vi "ServerVI.vi"() -> ()   [LabVIEW 2021]
uses:
  Resources/ServerEnum.ctl
  <vilib>/Utility/error.llb/DialogType.ctl
  <vilib>/Utility/file.llb/Read Delimited Spreadsheet (string).vi
  <vilib>/Utility/file.llb/Write Delimited Spreadsheet (string).vi
panel:
  in  "CarWashRecord":enum32{"Car Wash Record", "Revenue"}(tab)
  in  "btnLogout":bool
  out "Car Wash Record":string[][](table)
  out "Deluxe":dbl
  out "Economy":dbl
  in  "btnGenerate":bool
  out "Date":string
  out "Revenue ($)":dbl
  in  "LoginTab":enum32{"Login"}(tab)
  in  "Username":string
  in  "Password":string
  in  "btnLogin":bool
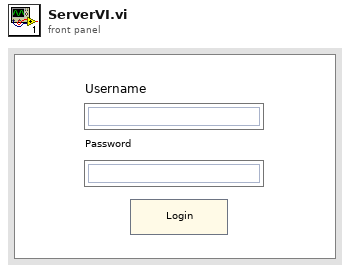
[diagram p1: front panel]
types:
  T1 = typedef "DialogType.ctl" = u16
  T2 = typedef "ServerEnum.ctl" = enum16{"Initialization", "Setup", "Validation", "ShowUI", "Format", "Error"}
  T3 = enum8{"Enabled", "Disabled", "Disabled and Grayed Out"}
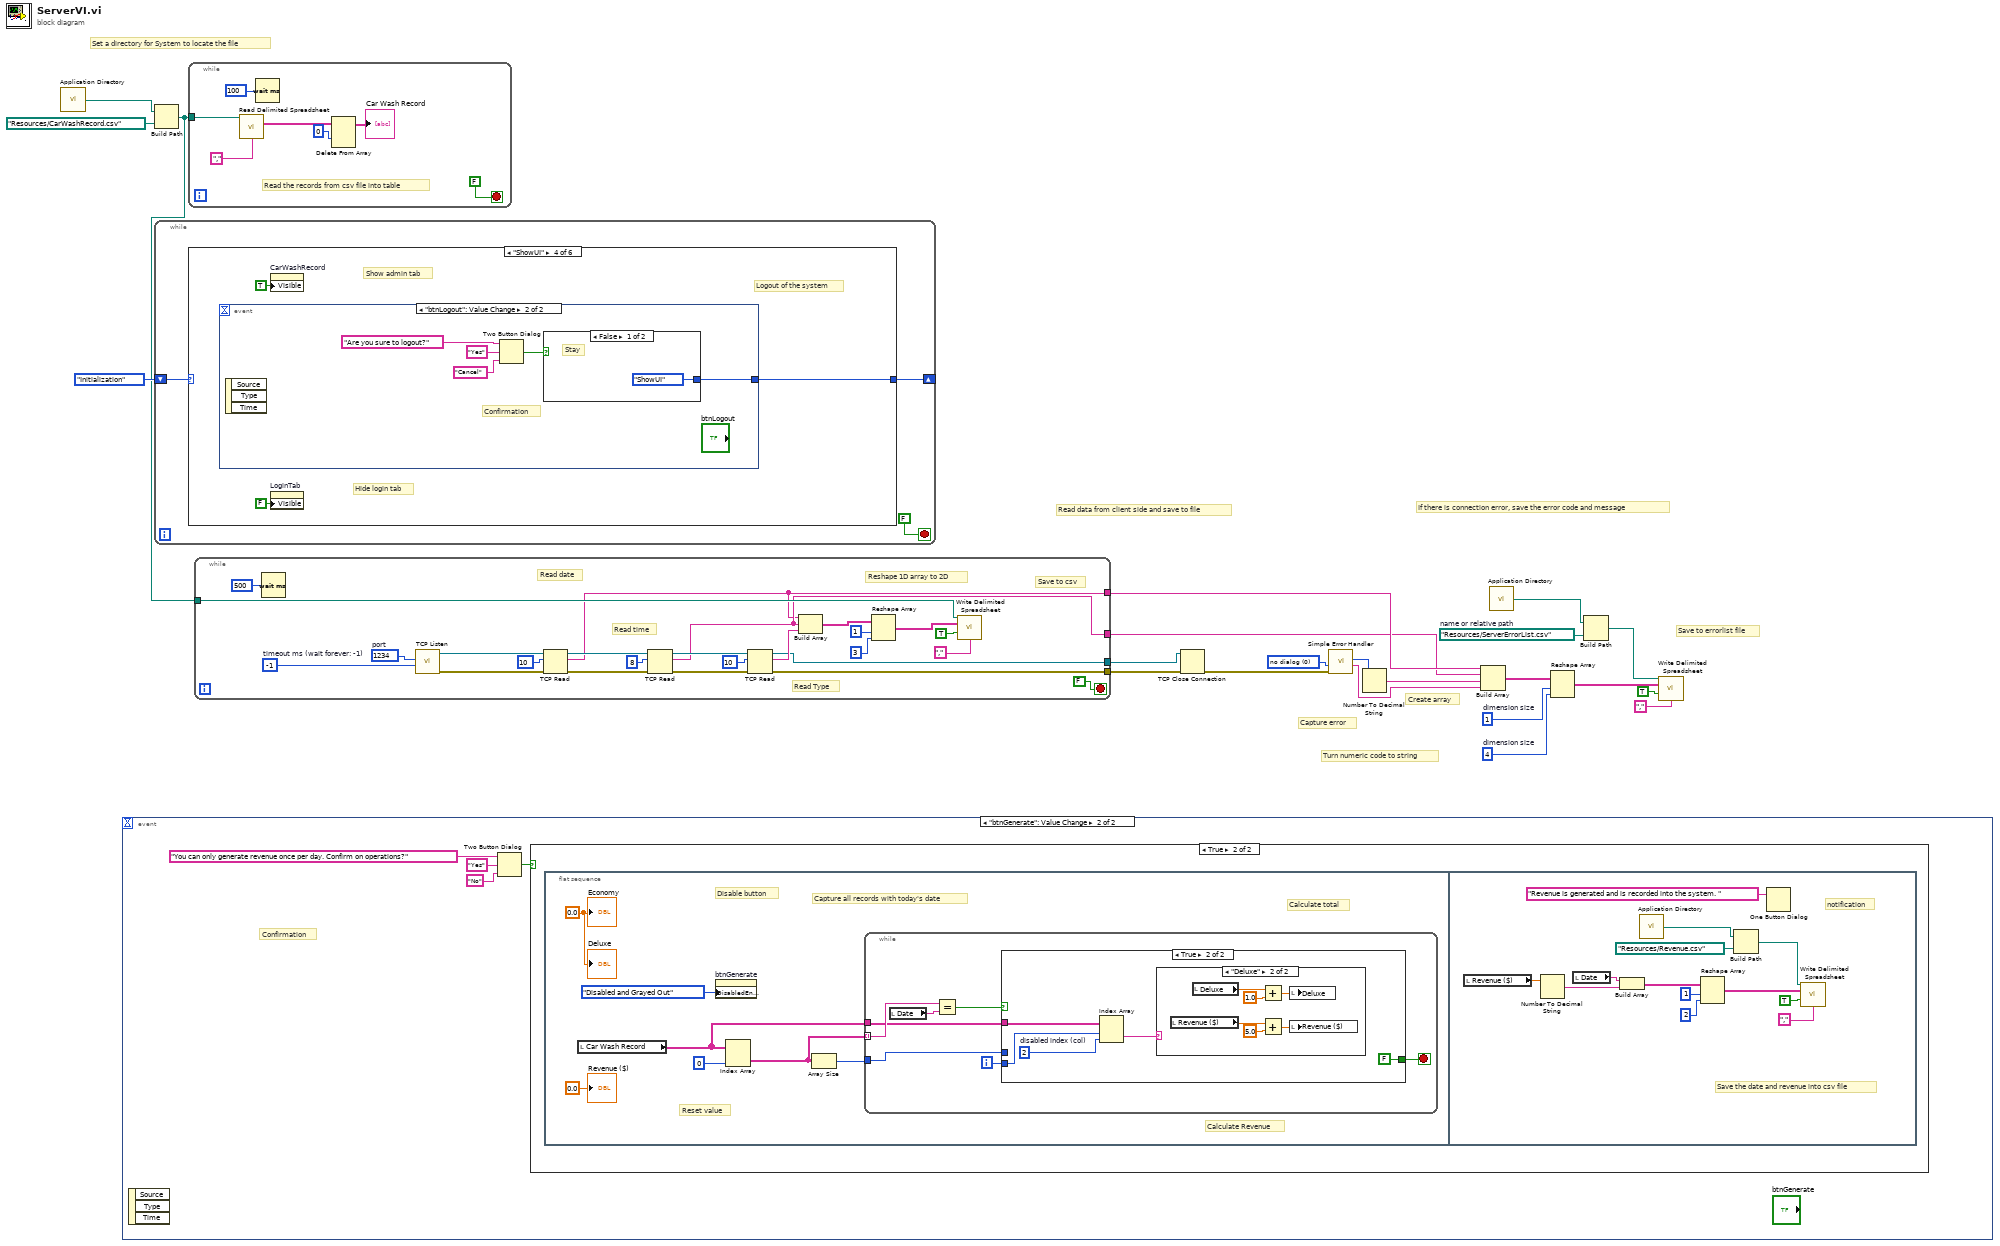
[diagram p0: block diagram]
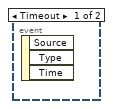
[diagram p2: hidden frame]
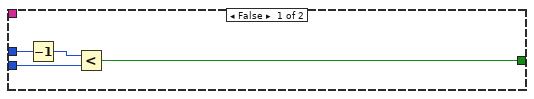
[diagram p4: hidden frame]
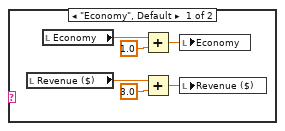
[diagram p5: hidden frame]
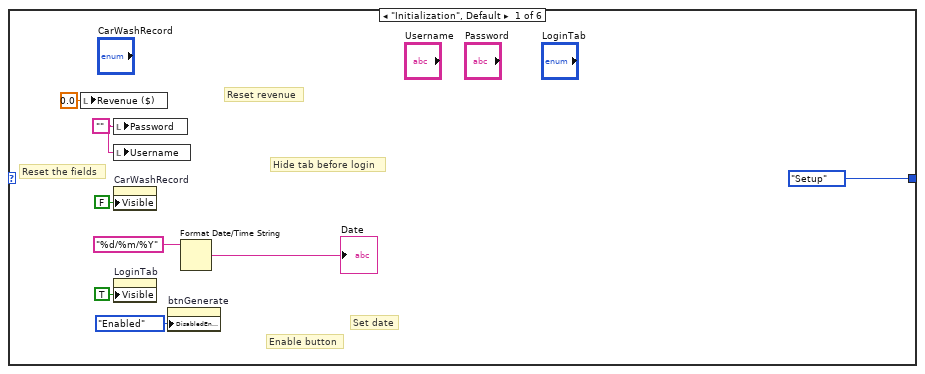
[diagram p6: hidden frame]
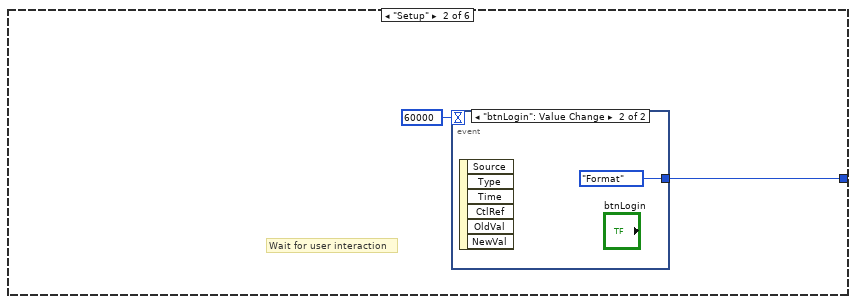
[diagram p7: hidden frame]
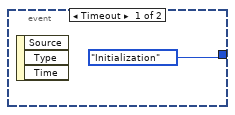
[diagram p8: hidden frame]
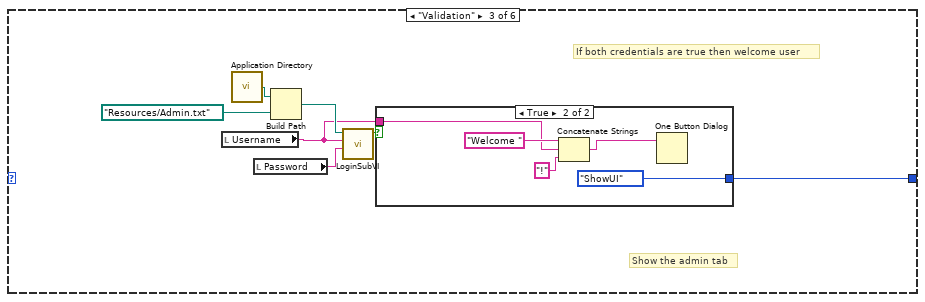
[diagram p9: hidden frame]
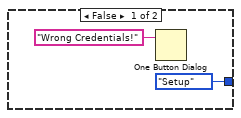
[diagram p10: hidden frame]
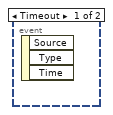
[diagram p11: hidden frame]
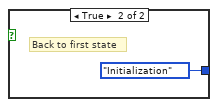
[diagram p12: hidden frame]
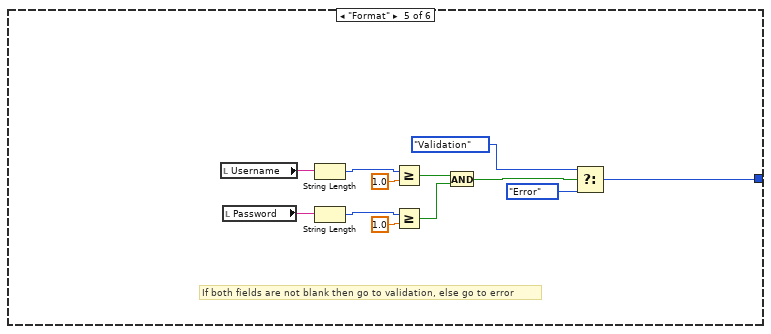
[diagram p13: hidden frame]
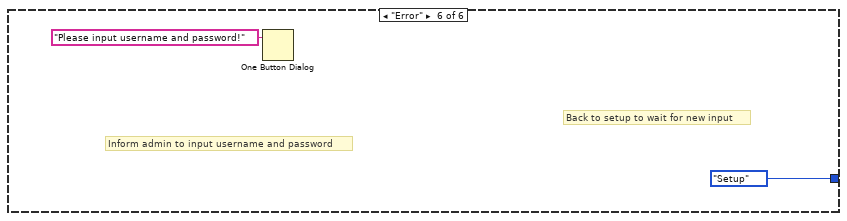
[diagram p14: hidden frame]
diagram:
  w6 = T1 0 items=["no dialog", "OK message", "continue or stop message", "OK message + warnings", "continue/stop + warnings"] ("type of dialog (OK msg:1)")
  w8 = 4  # dimension size
  w9 = 1  # dimension size
  w16 = path "Resources/ServerErrorList.csv"  # name or relative path
  # "If there is connection error, save the error code and message"
  # "Read data from client side and save to file"
  # "Create array"
  # "Turn numeric code to string"
  # "Capture error"
  # "Save to errorlist file"
  # "Set a directory for System to locate the file"
  n1 = call <vilib>:"Application Directory.vi"() -> ("Application Directory"=w20:path)
  n2 = event shown="[1] \"btnGenerate\": Value Change" {
    selector: _ -> [_ _]
    dyn-events: _ -> [_ _]
    timeout: _ -> [_ _]
    event Timeout {
      n3 = event-data() -> ()  [unwired: 1 in, 3 out]
    }
    event "btnGenerate": Value Change {
      # "Confirmation"
      n4 = event-data() -> ()  [unwired: 1 in, 3 out]
      n5 = Two Button Dialog(message="You can only generate revenue once per day. Confirm on operations?", 1:"No" ("F button name (\"Cancel\")"), 2:"Yes" ("T button name (\"OK\")")) -> (T button?=w23:bool)
      n6 = case shown="True" w23 {
        frame False {
        }
        frame True {
          n7 = flat-sequence {
            frame #0 {
              w27 = 0.0 ("Economy")
              # "Reset value"
              # "Calculate total"
              # "Calculate Revenue"
              # "Capture all records with today's date"
              # "Disable button"
              n8 = local read "Car Wash Record"() -> (w31:string[][])
              n9 = property on="btnGenerate" class="Bool (strict)"("DisabledEnum"=T3."Disabled and Grayed Out" ("Disabled")) -> ()  [unwired: 2 in, 2 out]
              n10 = Index Array "Index Array"(array=w31, index (col)=0 ("disabled index (col)")) -> (element=w29:string[])  [unwired: 1 in]
              n11 = Array Size(array=w29) -> (size(s)=w30:i32)
              n12 = while {
                tunnel: w30 -> [w37]
                tunnel: w29 -> [w40] mode=indexing
                tunnel: w31 -> [w38]
                i -> [w36]
                stop <- w34 stop-if-true
                n13 = local read "Date"() -> (w35:string)
                n14 = Equal?(x=w40, y=w35) -> (x = y?=w39:bool)
                n15 = case shown="True" w39 {
                  tunnel: w38 -> [_ w49]
                  tunnel: w37 -> [w43 _]
                  tunnel: w36 -> [w42 w48]
                  tunnel: [w41 FALSE] -> w34
                  frame False {
                    n16 = Decrement(x=w43) -> (x-1=w44:i32)
                    n17 = Less?(x=w44, y=w42) -> (x < y?=w41:bool)
                  }
                  frame True {
                    w47 = 2  # disabled index (col)
                    n18 = Index Array "Index Array"(array=w49, index (row)=w48, index (col)=w47) -> (element=w46:string)
                    n19 = case shown="\"Deluxe\"" w46 {
                      frame "Economy", Default {
                        n20 = local read "Revenue ($)"() -> (w55:dbl)
                        n21 = local read "Economy"() -> (w51:dbl)
                        n22 = Add(x=w51, y=1.0) -> (x+y=w52:dbl)
                        n23 = Add(x=w55, y=3.0) -> (x+y=w53:dbl)
                        n24 = local write "Economy"(w52) -> ()
                        n25 = local write "Revenue ($)"(w53) -> ()
                      }
                      frame "Deluxe" {
                        n26 = local read "Revenue ($)"() -> (w61:dbl)
                        n27 = local read "Deluxe"() -> (w58:dbl)
                        n28 = Add(x=w58, y=1.0) -> (x+y=w56:dbl)
                        n29 = Add(x=w61, y=5.0) -> (x+y=w60:dbl)
                        n30 = local write "Deluxe"(w56) -> ()
                        n31 = local write "Revenue ($)"(w60) -> ()
                      }
                    }
                  }
                }
              }
              "Revenue ($)" <- 0.0 ("Revenue")
              "Economy" <- w27
              "Deluxe" <- w27
            }
            frame #1 {
              # "notification"
              # "Save the date and revenue into csv file"
              n32 = local read "Revenue ($)"() -> (w70:dbl)
              n33 = Number To Decimal String(number=w70) -> (decimal integer string=w71:string)  [unwired: 1 in]
              n34 = local read "Date"() -> (w69:string)
              n35 = Build Array "Build Array"(w69, w71) -> (w72:string[])
              n36 = call <vilib>:"Application Directory.vi"() -> ("Application Directory"=w68:path)
              n37 = Reshape Array "Reshape Array"(w72, 1 ("dimension size"), 2 ("dimension size")) -> (w74:string[][])
              n38 = Build Path(base path=w68, name or relative path=path "Resources/Revenue.csv") -> (appended path=w73:path)
              n39 = One Button Dialog(message="Revenue is generated and is recorded into the system. ") -> ()  [unwired: 1 in, 1 out]
              n40 = call-poly <vilib>:"Write Delimited Spreadsheet.vi"("file path (dialog if empty)"=w73, "2D data"=w74, "append to file? (new file:F)"=TRUE, "delimiter (\\t)"="," ("delimiter (\\t)")) -> ()  [unwired: 10 in, 2 out]
            }
          }
        }
      }
    }
  }
  n41 = Build Path(base path=w20, name or relative path=path "Resources/CarWashRecord.csv") -> (appended path=w1:path)
  n42 = while {
    shift-right: [w76] -> _
    shift-left: ServerEnum."Initialization" -> [w77]
    stop <- FALSE stop-if-true
    n43 = case shown="\"ShowUI\"" w77 {
      tunnel: [ServerEnum."Setup" w87 w94 w104 w114 ServerEnum."Setup"] -> w76
      frame "Initialization", Default {
        w83 = ""
        # "Enable button"
        # "Set date"
        # "Reset revenue"
        # "Reset the fields"
        # "Hide tab before login"
        n44 = local write "Revenue ($)"(0.0 ("Revenue")) -> ()
        n45 = local write "Password"(w83) -> ()
        n46 = local write "Username"(w83) -> ()
        n47 = property on="CarWashRecord" class="TabCtl (strict)"("Visible"=FALSE) -> ()  [unwired: 2 in, 2 out]
        n48 = property on="LoginTab" class="TabCtl (strict)"("Visible"=TRUE) -> ()  [unwired: 2 in, 2 out]
        n49 = property on="btnGenerate" class="Bool (strict)"("DisabledEnum"=T3."Enabled" ("Disabled")) -> ()  [unwired: 2 in, 2 out]
        n50 = Format Date/Time String(time format string (%c)="%d/%m/%Y") -> (date/time string=→"Date":string)  [unwired: 2 in]
      }
      frame "Setup" {
        # "Wait for user interaction"
        n51 = event shown="[1] \"btnLogin\": Value Change" {
          selector: _ -> [_ _]
          dyn-events: _ -> [_ _]
          timeout: 60000 -> [_ _]
          tunnel: [ServerEnum."Initialization" ServerEnum."Format"] -> w87
          event Timeout {
            n52 = event-data() -> ()  [unwired: 1 in, 3 out]
          }
          event "btnLogin": Value Change {
            n53 = event-data() -> ()  [unwired: 1 in, 6 out]
          }
        }
      }
      frame "Validation" {
        # "Show the admin tab"
        # "If both credentials are true then welcome user"
        n54 = local read "Username"() -> (w90:string)
        n55 = call <vilib>:"Application Directory.vi"() -> ("Application Directory"=w93:path)
        n56 = local read "Password"() -> (w96:string)
        n57 = Build Path(base path=w93, name or relative path=path "Resources/Admin.txt") -> (appended path=w91:path)
        n58 = call "LoginSubVI.vi"("Password"=w96, "Username"=w90, "file path (dialog if empty)"=w91) -> ("Status"=w95:bool)  [unwired: 8 in]
        n59 = case shown="True" w95 {
          tunnel: [ServerEnum."Setup" ServerEnum."ShowUI"] -> w94
          tunnel: w90 -> [_ w101]
          frame False {
            n60 = One Button Dialog(message="Wrong Credentials!") -> ()  [unwired: 1 in, 1 out]
          }
          frame True {
            n61 = Concatenate Strings("Welcome " ("message"), w101, "!" ("string")) -> (w100:string)
            n62 = One Button Dialog(message=w100) -> ()  [unwired: 1 in, 1 out]
          }
        }
      }
      frame "ShowUI" {
        # "Show admin tab"
        # "Hide login tab"
        # "Logout of the system"
        n63 = event shown="[1] \"btnLogout\": Value Change" {
          selector: _ -> [_ _]
          dyn-events: _ -> [_ _]
          timeout: _ -> [_ _]
          tunnel: [_ w111] -> w104
          event Timeout {
            n64 = event-data() -> ()  [unwired: 1 in, 3 out]
          }
          event "btnLogout": Value Change {
            # "Confirmation"
            n65 = event-data() -> ()  [unwired: 1 in, 3 out]
            n66 = Two Button Dialog(message="Are you sure to logout?", 1:"Cancel" ("F button name (\"Cancel\")"), 2:"Yes" ("T button name (\"OK\")")) -> (T button?=w107:bool)
            n67 = case shown="False" w107 {
              tunnel: [ServerEnum."ShowUI" ServerEnum."Initialization"] -> w111
              frame False {
                # "Stay"
              }
              frame True {
                # "Back to first state"
              }
            }
          }
        }
        n68 = property on="CarWashRecord" class="TabCtl (strict)"("Visible"=TRUE) -> ()  [unwired: 2 in, 2 out]
        n69 = property on="LoginTab" class="TabCtl (strict)"("Visible"=FALSE) -> ()  [unwired: 2 in, 2 out]
      }
      frame "Format" {
        # "If both fields are not blank then go to validation, else go to error"
        n70 = local read "Username"() -> (w117:string)
        n71 = local read "Password"() -> (w118:string)
        n72 = String Length(string=w117) -> (length=w124:i32)
        n73 = String Length(string=w118) -> (length=w122:i32)
        n74 = Greater Or Equal?(x=w124, y=1.0) -> (x >= y?=w119:bool)
        n75 = Greater Or Equal?(x=w122, y=1.0) -> (x >= y?=w121:bool)
        n76 = And(x=w119, y=w121) -> (x .and. y?=w120:bool)
        n77 = Select(t=ServerEnum."Validation", s=w120, f=ServerEnum."Error") -> (s? t:f=w114:T2)
      }
      frame "Error" {
        # "Back to setup to wait for new input"
        # "Inform admin to input username and password"
        n78 = One Button Dialog(message="Please input username and password!") -> ()  [unwired: 1 in, 1 out]
      }
    }
  }
  n79 = while {
    tunnel: w1 -> [w131]
    stop <- FALSE stop-if-true
    # "Read the records from csv file into table"
    n80 = call-poly <vilib>:"Read Delimited Spreadsheet.vi"("file path (dialog if empty)"=w131, "delimiter (\\t)"="," ("delimiter (\\t)")) -> ("all rows"=w130:string[][])  [unwired: 8 in, 5 out]
    n81 = Wait (ms)(milliseconds to wait=u32 100) -> ()  [unwired: 1 out]
    n82 = Delete From Array(array=w130, index (row)=0) -> (array with subset deleted=→"Car Wash Record":string[][])  [unwired: 2 in, 1 out]
  }
  n83 = while {
    tunnel: [w145] -> w22
    tunnel: [w135] -> w21
    tunnel: w1 -> [w138]
    tunnel: [w136] -> w3
    tunnel: [w137] -> w2
    stop <- FALSE stop-if-true
    w158 = -1  # timeout ms (wait forever: -1)
    w159 = u16 1234  # port
    # "Save to csv"
    # "Reshape 1D array to 2D"
    # "Read Type"
    # "Read time"
    # "Read date"
    n84 = Wait (ms)(milliseconds to wait=u32 500) -> ()  [unwired: 1 out]
    n85 = call <vilib>:"TCP Listen.vi"("timeout ms (wait forever: -1)"=w158, "port"=w159) -> ("error out"=w156:errorcluster, "connection ID"=w157:refnum<k5>)  [unwired: 5 in, 3 out]
    n86 = TCP Read(connection ID=w157, bytes to read=10, error in (no error)=w156) -> (connection ID out=w155:refnum<k5>, data out=w136:string, error out=w154:errorcluster)  [unwired: 2 in]
    n87 = TCP Read(connection ID=w155, bytes to read=8, error in (no error)=w154) -> (connection ID out=w153:refnum<k5>, data out=w137:string, error out=w152:errorcluster)  [unwired: 2 in]
    n88 = TCP Read(connection ID=w153, bytes to read=10, error in (no error)=w152) -> (connection ID out=w135:refnum<k5>, data out=w150:string, error out=w145:errorcluster)  [unwired: 2 in]
    n89 = Build Array "Build Array"(w136, w137, w150) -> (w144:string[])
    n90 = Reshape Array "Reshape Array"(w144, 1 ("dimension size"), 3 ("dimension size")) -> (w139:string[][])
    n91 = call-poly <vilib>:"Write Delimited Spreadsheet.vi"("file path (dialog if empty)"=w138, "2D data"=w139, "append to file? (new file:F)"=TRUE, "delimiter (\\t)"="," ("delimiter (\\t)")) -> ()  [unwired: 10 in, 2 out]
  }
  n92 = TCP Close Connection(connection ID=w21, error in (no error)=w22) -> (error out=w4:errorcluster)  [unwired: 1 in, 1 out]
  n93 = call <vilib>:"Simple Error Handler.vi"("type of dialog (OK msg:1)"=w6, "error in (no error)"=w4) -> ("code out"=w12:i32, "source out"=w5:string)  [unwired: 3 in, 3 out]
  n94 = Number To Decimal String(number=w12) -> (decimal integer string=w11:string)  [unwired: 1 in]
  n95 = Build Array "Build Array"(w3, w2, w11, w5) -> (w10:string[])
  n96 = call <vilib>:"Application Directory.vi"() -> ("Application Directory"=w17:path)
  n97 = Reshape Array "Reshape Array"(w10, w9, w8) -> (w7:string[][])
  n98 = Build Path(base path=w17, name or relative path=w16) -> (appended path=w15:path)
  n99 = call-poly <vilib>:"Write Delimited Spreadsheet.vi"("file path (dialog if empty)"=w15, "2D data"=w7, "append to file? (new file:F)"=TRUE, "delimiter (\\t)"="," ("delimiter (\\t)")) -> ()  [unwired: 10 in, 2 out]
